vi "SynapseAPI-Get Tank.vi"(0 "URL":string="http://localhost:24414", 11 "error in (no error)":errorcluster) -> (8 "tank":string, 15 "error out":errorcluster)   [LabVIEW 2020]
uses:
  <vilib>/httpClient/LabVIEWHTTPClient.lvlib
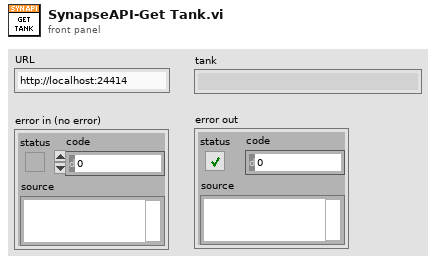
[diagram p1: front panel]
types:
  T1 = typedef "LabVIEWHTTPClient.lvlib/ClientHandle.ctl" = refnum<k1>
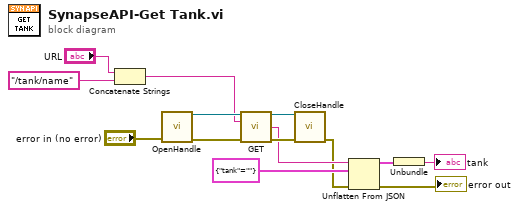
[diagram p0: block diagram]
diagram:
  n1 = Concatenate Strings("URL", "/tank/name") -> (w8:string)
  n2 = call <vilib>:"OpenHandle.vi"("error in (no error)"="error in (no error)") -> ("client handle out"=w11:T1, "error out"=w10:errorcluster)  [unwired: 13 in]
  n3 = call <vilib>:"GET.vi"("client handle"=w11, "url"=w8, "error in (no error)"=w10) -> ("client handle out"=w13:T1, "body"=w7:string, "error out"=w14:errorcluster)  [unwired: 9 in, 1 out]
  n4 = call <vilib>:"CloseHandle.vi"("client handle"=w13, "error in (no error)"=w14) -> ("error out"=w4:errorcluster)  [unwired: 13 in]
  n5 = Unflatten From JSON(JSON string=w7, type and defaults=cluster{"tank":string} {"tank"=""} ("Cluster"), error in (no error)=w4) -> (value=w2:cluster{"tank":string}, error out=→"error out":errorcluster)  [unwired: 4 in]
  n6 = Unbundle(w2) -> ("tank"=→"tank":string)
